vi "GviewerMain.vi"() -> ()   [LabVIEW 2020, in "Gviewer.lvclass"]
doc: "Main Graph Viewer.\nSeveral instances of this viewer can run simultaneously."
uses:
  Gviewer.lvclass
  controls/Typedef_Live.ctl
  Gserver/controls/Typedef_Gviewer-Query.ctl
  Gserver/controls/Typedef_QueryType.ctl
  Gviewer.lvclass/Gviewer.ctl
  FAMM/controls/FAMM_reply_datagram.ctl
  FAMM/controls/FAMM_reply_PAQdata.ctl
  FAMM/controls/FAMM_reply_WAQdata.ctl
  FAMM/controls/FAMM_reply_EAQdata.ctl
  controls/ToolBarAppearance.ctl
  controls/KeyPress.ctl
  <vilib>/event_ctls.llb/eventvkey.ctl
  Gserver/Gserver.lvclass
  FAMM/FAMM.lvclass
panel:
  in  "StartupTagList":string[](array[string])
  in  "Gserver-Queue":refnum<queue>
  in  "GviewName":string="Gview-01"
  in  "Live":T1
  out "ToolBar":picture
  out "Graph":cluster{dbl[], "data":dbl[]}[](graph)
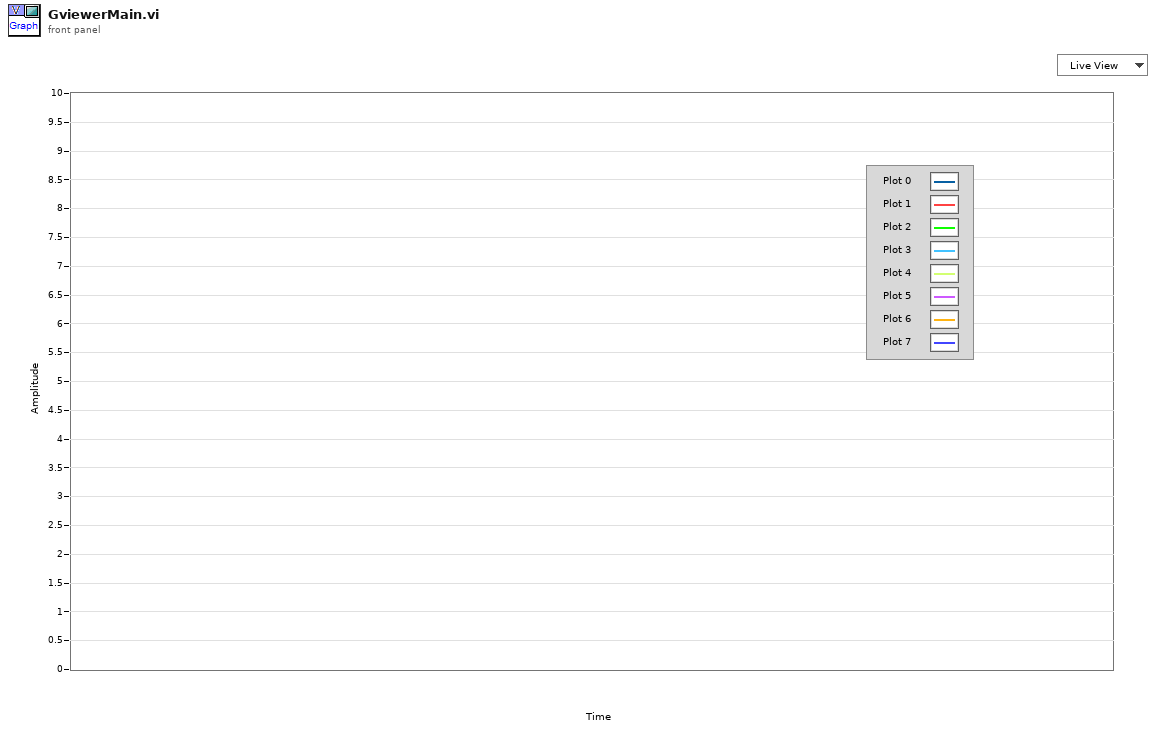
[diagram p1: front panel]
types:
  T1 = typedef "Gviewer.lvclass/Typedef_Live.ctl" = enum16{"Live View", "Freeze"}
  T2 = typedef "FAMM.lvclass/FAMM_reply_datagram.ctl" = cluster{"GraphName":string, "Time-Start":timestamp, "Time-End":timestamp, "TimeSpan":dbl, "Live":T1, "PAQ_section":T3, "WAQ_section":T4, "EAQ_section":T5}
  T3 = typedef "FAMM.lvclass/FAMM_reply_PAQdata.ctl" = cluster{"Tags":string[], "time stamp":timestamp[], "DataSection":cluster{"data":dbl[], "max":dbl[], "min":dbl[], "Status":u32[]}[]}
  T4 = typedef "FAMM.lvclass/FAMM_reply_WAQdata.ctl" = cluster{"Boolean":bool}
  T5 = typedef "FAMM.lvclass/FAMM_reply_EAQdata.ctl" = cluster{"Boolean":bool}
  T6 = typedef "Gserver.lvclass/Typedef_QueryType.ctl" = enum16{"Subscribe", "DataRequest", "RequestAllTags", "RequestIniPath", "FAMMstarted", "SetClientOptions", "GviewerUpdate", "OpenNewGraph", "CloseClient", "CloseAllClients", "Close Gserver"}
  T7 = typedef "Gviewer.lvclass/ToolBarAppearance.ctl" = enum16{"Bare", "Native", "Gradient"}
  T8 = typedef "KeyPress.ctl" = cluster{"Char":i16, "VKey":T9, "Shift":bool, "Ctrl":bool, "Time":timestamp}
  T9 = typedef "eventvkey.ctl" = enum16{"ASCII", "Enter", "Return", "Shift", "Ctrl", "Alt", "Cmd", "Opt", "Caps", "NumLock", "Clear", "Break", "Up", "Down", "Left", "Right", "Insert", "Delete", "Home", "End", "PageUp", "PageDown", "Escape", "Help", "Pause", "ScrollLock", "F1", "F2", "F3", "F4", "F5", "F6", "F7", "F8", "F9", "F10", "F11", "F12", "F13", "F14", "F15", "F16", "F17", "F18", "F19", "F20", "F21", "F22", "F23", "F24", "Play", "VolumeUp", "VolumeDown", "Mute", "Two Byte Char"}
  T10 = typedef "Typedef_Gserver-Replies.ctl" = cluster{"ServerActions":T11, "data":variant, "Source":string, "Time Stamp":timestamp}
  T11 = typedef "Typedef_ServerActions.ctl" = enum16{"GraphUpdate", "SendAllTags", "SendIniPath", "SetGeneralOptions", "ExitGraph"}
  T12 = typedef "SettingsGeneral.ctl" = cluster{"MenuBar_active":bool, "ContextMenu_active":bool}
  T13 = typedef "LVPoint32TypeDef.ctl" = cluster{"Horizontal":i32, "Vertical":i32}
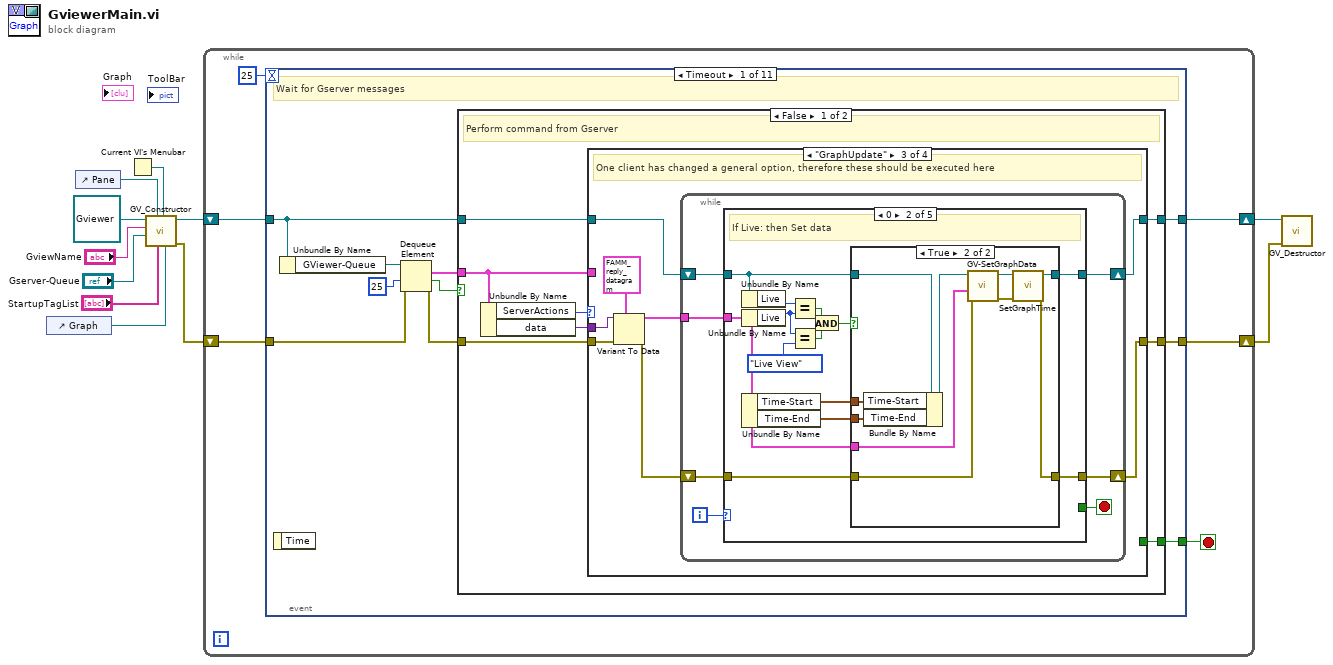
[diagram p0: block diagram]
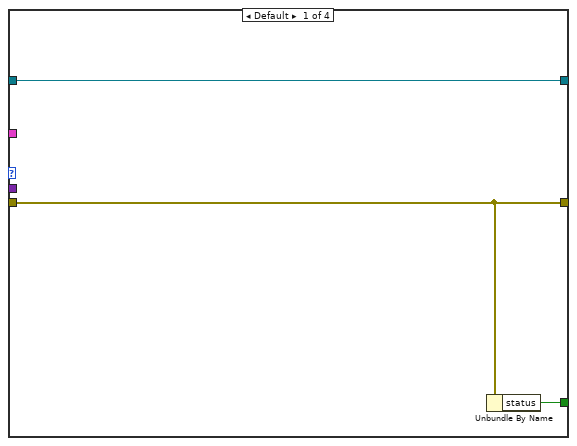
[diagram p2: hidden frame]
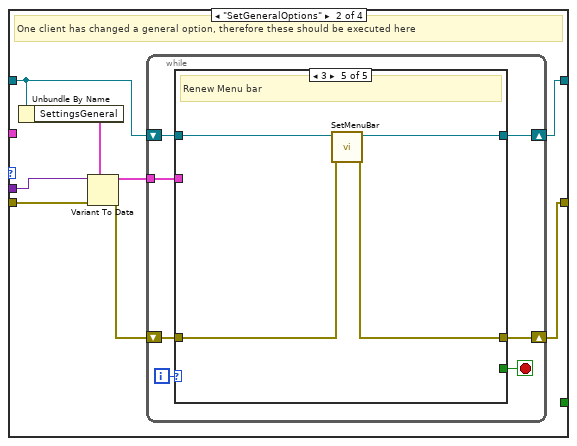
[diagram p3: hidden frame]
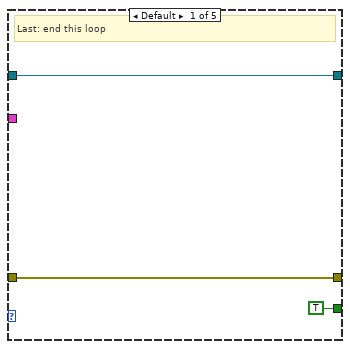
[diagram p4: hidden frame]
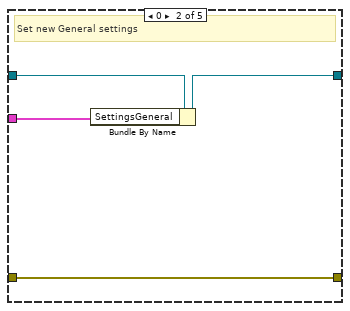
[diagram p5: hidden frame]
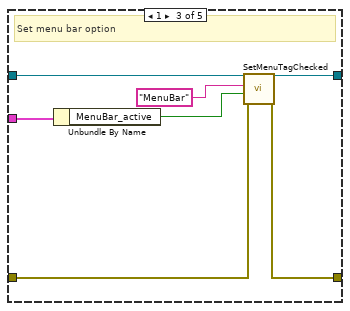
[diagram p6: hidden frame]
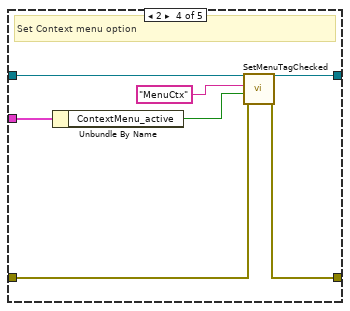
[diagram p7: hidden frame]
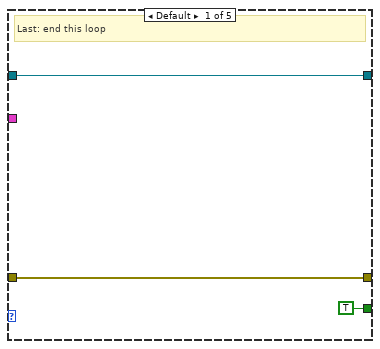
[diagram p8: hidden frame]
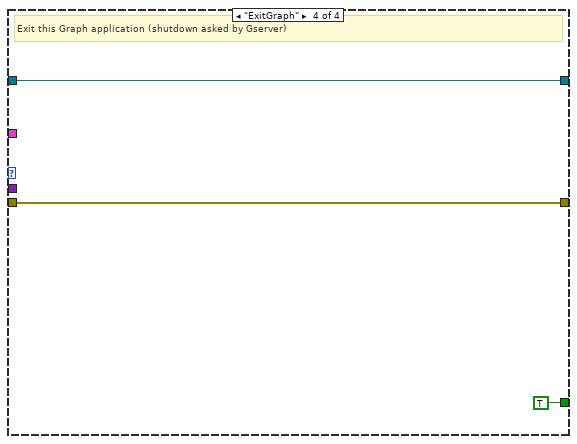
[diagram p13: hidden frame]
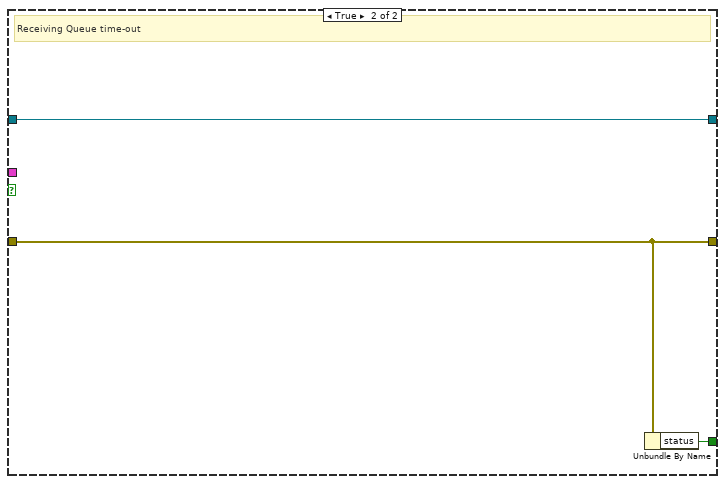
[diagram p14: hidden frame]
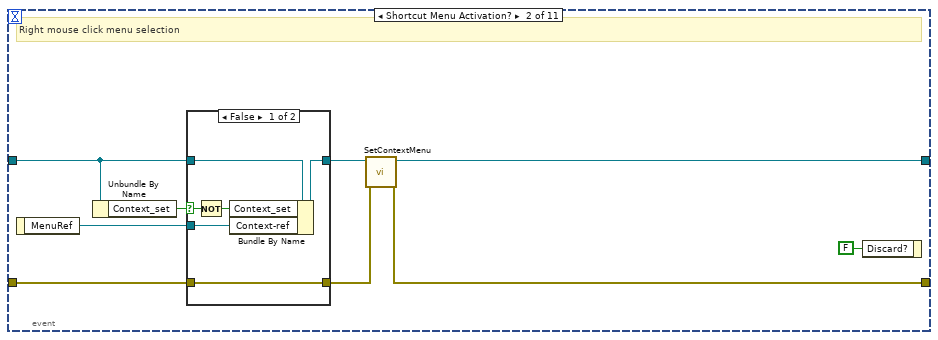
[diagram p15: hidden frame]
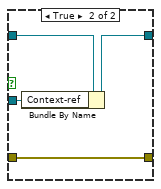
[diagram p16: hidden frame]
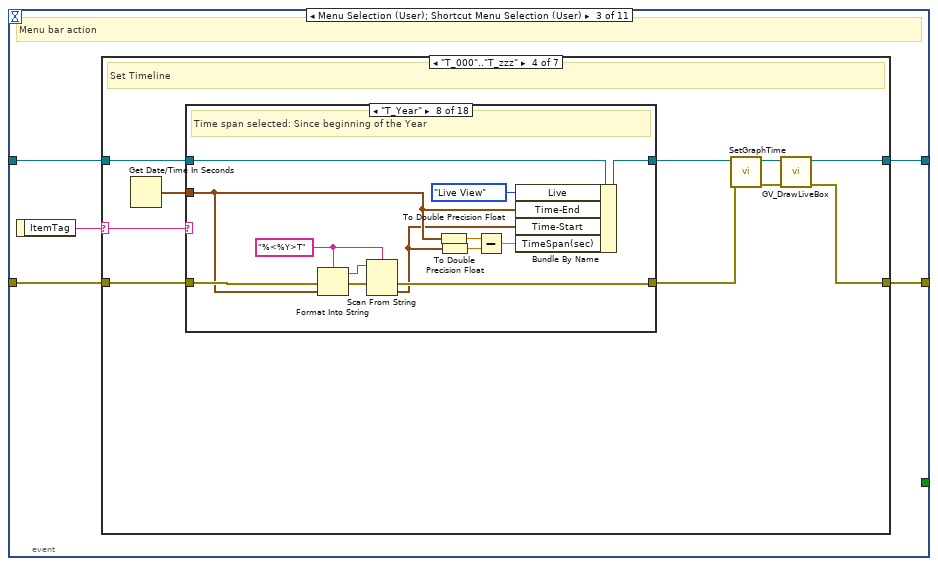
[diagram p17: hidden frame]
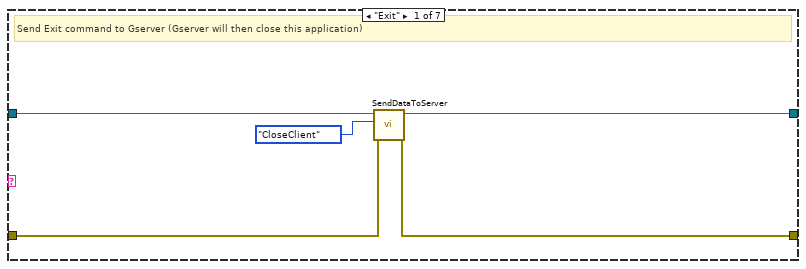
[diagram p18: hidden frame]
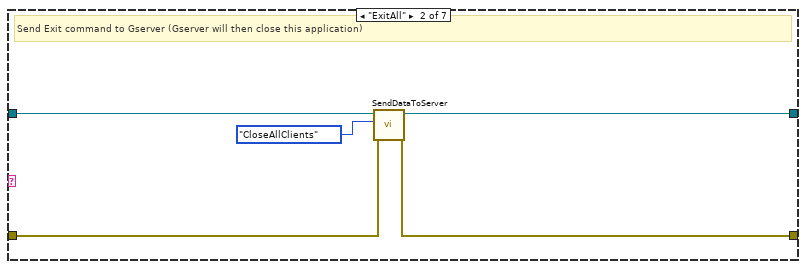
[diagram p19: hidden frame]
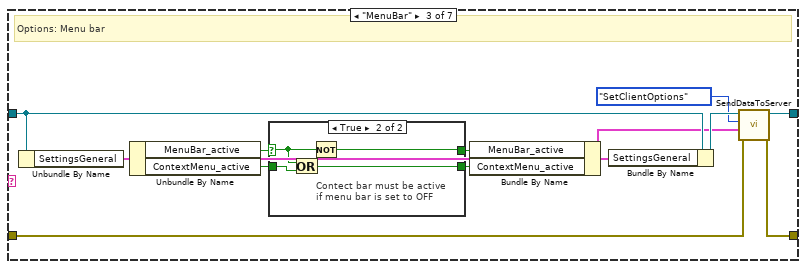
[diagram p20: hidden frame]
diagram:
  n1 = control-ref of="Graph"() -> (w1:refnum<vi>)
  n2 = control-ref of="Pane"() -> (w7:refnum<vi>)
  n3 = Current VI's Menubar() -> (w2:refnum<k9>)
  n4 = call "GV_Constructor.vi"("Graph-ref"=w1, "menu reference"=w2, "StartupTagList"="StartupTagList", "Pane"=w7, "Gserver-Queue"="Gserver-Queue", "GviewName"="GviewName", "Gviewer in"=refnum<class "Gviewer.lvclass"> refnum) -> ("error out"=w3:errorcluster, "Gviewer out"=w10:refnum<class "Gviewer.lvclass">)  [unwired: 3 in]
  n5 = while {
    shift-right: [w15] -> w11
    shift-left: w10 -> [w16]
    shift-right: [w13] -> w9
    shift-left: w3 -> [w14]
    stop <- w12 stop-if-true
    n6 = event shown="[0] Timeout" {
      selector: _ -> [_ _ _ _ _ _ _ _ _ _ _]
      dyn-events: _ -> [_ _ _ _ _ _ _ _ _ _ _]
      timeout: 25 -> [_ _ _ _ _ _ _ _ _ _ _]
      tunnel: w16 -> [w18 w141 w156 w396 w399 w411 w450 w471 w477 w484 w488]
      tunnel: [w21 w135 w154 w391 w397 w406 w444 w472 w475 w481 w487] -> w15
      tunnel: w14 -> [w26 w139 w155 w395 w400 w410 w449 w469 w473 w480 w485]
      tunnel: [w22 w137 w153 w389 w400 w404 w441 w470 w474 w479 w485] -> w13
      tunnel: [w20 _ _ _ _ _ _ _ _ _ _] -> w12
      event Timeout {
        # "Wait for Gserver messages"
        n7 = event-data() -> ()  [unwired: 1 in, 1 out]
        n8 = Unbundle By Name(w18) -> ("GViewer-Queue"=w27:refnum<queue>)
        n9 = Dequeue Element(queue=w27, timeout in ms (-1)=25, error in (no error)=w26) -> (element=w24:T10, timed out?=w19:bool, error out=w23:errorcluster)  [unwired: 1 out]
        n10 = case shown="False" w19 {
          tunnel: w24 -> [w29 _]
          tunnel: w18 -> [w34 w133]
          tunnel: w23 -> [w33 w132]
          tunnel: [w32 w132] -> w22
          tunnel: [w31 w133] -> w21
          tunnel: [w30 w131] -> w20
          frame False {
            # "Perform command from Gserver"
            n11 = Unbundle By Name(w29) -> ("ServerActions"=w35:T11, "data"=w28:variant)
            n12 = case shown="\"GraphUpdate\"" w35 {
              tunnel: w34 -> [w38 w40 w81 w130]
              tunnel: w33 -> [w36 w45 w85 w129]
              tunnel: [w36 w41 w82 w129] -> w32
              tunnel: [w38 w43 w84 w130] -> w31
              tunnel: [w37 _ _ TRUE] -> w30
              tunnel: w29 -> [_ _ _ _]
              tunnel: w28 -> [_ w46 w86 _]
              frame Default {
                n13 = Unbundle By Name(w36) -> ("status"=w37:bool)
              }
              frame "SetGeneralOptions" {
                # "One client has changed a general option, therefore these should be executed here"
                n14 = Unbundle By Name(w40) -> ("SettingsGeneral"=w44:T12)
                n15 = Variant To Data(error in=w45, type=w44, Variant=w46) -> (data=w39:T12, error out=w42:errorcluster)
                n16 = while {
                  shift-right: [w48] -> w43
                  shift-left: w40 -> [w51]
                  shift-right: [w47] -> w41
                  shift-left: w42 -> [w50]
                  tunnel: w39 -> [w49]
                  i -> [w53]
                  stop <- w52 stop-if-true
                  n17 = case shown="3" w53 {
                    tunnel: [TRUE _ _ _ _] -> w52
                    tunnel: w51 -> [w54 w60 w62 w73 w78]
                    tunnel: w50 -> [w55 w57 w64 w69 w76]
                    tunnel: w49 -> [_ w59 w61 w71 _]
                    tunnel: [w54 w58 w66 w72 w77] -> w48
                    tunnel: [w55 w57 w63 w68 w75] -> w47
                    frame Default {
                      # "Last: end this loop"
                    }
                    frame 0 {
                      # "Set new General settings"
                      n18 = Bundle By Name(cluster=w60, "SettingsGeneral"=w59) -> (w58:refnum<class "Gviewer.lvclass">)
                    }
                    frame 1 {
                      # "Set menu bar option"
                      n19 = Unbundle By Name(w61) -> ("MenuBar_active"=w65:bool)
                      n20 = call "SetMenuTagChecked.vi"("error in (no error)"=w64, "Checked"=w65, "TAG"="MenuBar", "Gviewer in"=w62) -> ("error out"=w63:errorcluster, "Gviewer out"=w66:refnum<class "Gviewer.lvclass">)  [unwired: 6 in]
                    }
                    frame 2 {
                      # "Set Context menu option"
                      n21 = Unbundle By Name(w71) -> ("ContextMenu_active"=w70:bool)
                      n22 = call "SetMenuTagChecked.vi"("error in (no error)"=w69, "Checked"=w70, "TAG"="MenuCtx", "Gviewer in"=w73) -> ("error out"=w68:errorcluster, "Gviewer out"=w72:refnum<class "Gviewer.lvclass">)  [unwired: 6 in]
                    }
                    frame 3 {
                      # "Renew Menu bar"
                      n23 = call "SetMenuBar.vi"("error in (no error)"=w76, "Gviewer in"=w78) -> ("error out"=w75:errorcluster, "Gviewer out"=w77:refnum<class "Gviewer.lvclass">)  [unwired: 8 in]
                    }
                  }
                }
              }
              frame "GraphUpdate" {
                # "One client has changed a general option, therefore these should be executed here"
                n24 = Variant To Data(error in=w85, type=T2 {"GraphName"="", "Time-Start"=timestamp(0 s since 1904-01-01), "Time-End"=timestamp(0 s since 1904-01-01), "TimeSpan"=0.0, "Live"=enum."Live View", "PAQ_section"={"Tags"=[], "time stamp"=[], "DataSection"=[]}, "WAQ_section"={"Boolean"=FALSE}, "EAQ_section"={"Boolean"=FALSE}} ("GviewerUpdate"), Variant=w86) -> (data=w80:T2, error out=w83:errorcluster)
                n25 = while {
                  shift-right: [w88] -> w84
                  shift-left: w81 -> [w91]
                  shift-right: [w87] -> w82
                  shift-left: w83 -> [w90]
                  tunnel: w80 -> [w89]
                  i -> [w93]
                  stop <- w92 stop-if-true
                  n26 = case shown="0" w93 {
                    tunnel: [TRUE _ _ _ _] -> w92
                    tunnel: w91 -> [w94 w103 w123 w125 w127]
                    tunnel: w90 -> [w95 w101 w122 w124 w126]
                    tunnel: w89 -> [_ w97 _ _ _]
                    tunnel: [w94 w102 w123 w125 w127] -> w88
                    tunnel: [w95 w100 w122 w124 w126] -> w87
                    frame Default {
                      # "Last: end this loop"
                    }
                    frame 0 {
                      # "If Live: then Set data"
                      n27 = Unbundle By Name(w103) -> ("Live"=w109:T1)
                      n28 = Unbundle By Name(w97) -> ("Live"=w108:T1)
                      n29 = Unbundle By Name(w97) -> ("Time-Start"=w99:timestamp, "Time-End"=w98:timestamp)
                      n30 = Equal?(x=w109, y=w108) -> (x = y?=w106:bool)
                      n31 = Equal?(x=w108, y=Typedef_Live."Live View") -> (x = y?=w105:bool)
                      n32 = And(x=w106, y=w105) -> (x .and. y?=w104:bool)
                      n33 = case shown="True" w104 {
                        tunnel: w103 -> [w111 w119]
                        tunnel: [w111 w118] -> w102
                        tunnel: w101 -> [w110 w113]
                        tunnel: [w110 w117] -> w100
                        tunnel: w99 -> [_ w121]
                        tunnel: w98 -> [_ w120]
                        tunnel: w97 -> [_ w112]
                        frame False {
                        }
                        frame True {
                          n34 = Bundle By Name(cluster=w119, "Time-Start"=w121, "Time-End"=w120) -> (w116:refnum<class "Gviewer.lvclass">)
                          n35 = call "GV-SetGraphData.vi"("error in (no error)"=w113, "GviewerUpdate"=w112, "Gviewer in"=w116) -> ("error out"=w114:errorcluster, "Gviewer out"=w115:refnum<class "Gviewer.lvclass">)  [unwired: 7 in]
                          n36 = call "SetGraphTime.vi"("error in (no error)"=w114, "Gviewer in"=w115) -> ("error out"=w117:errorcluster, "Gviewer out"=w118:refnum<class "Gviewer.lvclass">)  [unwired: 8 in]
                        }
                      }
                    }
                    frame 1 {
                      # "1"
                    }
                    frame 2 {
                      # "2"
                    }
                    frame 3 {
                      # "3"
                    }
                  }
                }
              }
              frame "ExitGraph" {
                # "Exit this Graph application (shutdown asked by Gserver)"
              }
            }
          }
          frame True {
            # "Receiving Queue time-out"
            n37 = Unbundle By Name(w132) -> ("status"=w131:bool)
          }
        }
      }
      event Shortcut Menu Activation? {
        # "Right mouse click menu selection"
        n38 = event-data() -> ("MenuRef"=w140:refnum<k9>)  [unwired: 1 in]
        n39 = Unbundle By Name(w141) -> ("Context_set"=w142:bool)
        n40 = case shown="False" w142 {
          selector: w142 -> [w148 _]
          tunnel: w141 -> [w145 w149]
          tunnel: w140 -> [w146 w151]
          tunnel: w139 -> [w143 w152]
          tunnel: [w143 w152] -> w136
          tunnel: [w144 w150] -> w138
          frame False {
            n41 = Not(x=w148) -> (.not. x?=w147:bool)
            n42 = Bundle By Name(cluster=w145, "Context_set"=w147, "Context-ref"=w146) -> (w144:refnum<class "Gviewer.lvclass">)
          }
          frame True {
            n43 = Bundle By Name(cluster=w149, "Context-ref"=w151) -> (w150:refnum<class "Gviewer.lvclass">)
          }
        }
        n44 = call "SetContextMenu.vi"("error in (no error)"=w136, "Gviewer in"=w138) -> ("error out"=w137:errorcluster, "Gviewer out"=w135:refnum<class "Gviewer.lvclass">)  [unwired: 8 in]
        n45 = event-data("Discard?"=FALSE) -> ()  [unwired: 1 in, 1 out]
      }
      event Menu Selection (User); Shortcut Menu Selection (User) {
        # "Menu bar action"
        n46 = event-data() -> ("ItemTag"=w157:string)  [unwired: 1 in]
        n47 = case shown="\"T_000\"..\"T_zzz\"" w157 {
          selector: w157 -> [_ _ _ w196 _ w377 w387]
          tunnel: w156 -> [w161 w166 w176 w194 w360 w375 w388]
          tunnel: w155 -> [w160 w165 w170 w193 w357 w378 w384]
          tunnel: [w162 w167 w172 w189 w359 w380 w388] -> w154
          tunnel: [w159 w164 w171 w187 w358 w379 w384] -> w153
          frame "Exit" {
            # "Send Exit command to Gserver (Gserver will then close this application)"
            n48 = call "SendDataToServer.vi"("error in (no error)"=w160, "Query_type"=Typedef_QueryType."CloseClient", "Gviewer in"=w161) -> ("error out"=w159:errorcluster, "Gviewer out"=w162:refnum<class "Gviewer.lvclass">)  [unwired: 7 in]
          }
          frame "ExitAll" {
            # "Send Exit command to Gserver (Gserver will then close this application)"
            n49 = call "SendDataToServer.vi"("error in (no error)"=w165, "Query_type"=Typedef_QueryType."CloseAllClients", "Gviewer in"=w166) -> ("error out"=w164:errorcluster, "Gviewer out"=w167:refnum<class "Gviewer.lvclass">)  [unwired: 7 in]
          }
          frame "MenuBar" {
            # "Options: Menu bar"
            n50 = Unbundle By Name(w176) -> ("SettingsGeneral"=w178:T12)
            n51 = Unbundle By Name(w178) -> ("MenuBar_active"=w179:bool, "ContextMenu_active"=w175:bool)
            n52 = case shown="True" w179 {
              selector: w179 -> [w182 w184]
              tunnel: [w181 w186] -> w177
              tunnel: w175 -> [w180 w185]
              tunnel: [w180 w183] -> w174
              frame False {
                n53 = Not(x=w182) -> (.not. x?=w181:bool)
              }
              frame True {
                # "Contect bar must be active\nif menu bar is set to OFF"
                n54 = Or(x=w184, y=w185) -> (x .or. y?=w183:bool)
                n55 = Not(x=w184) -> (.not. x?=w186:bool)
              }
            }
            n56 = Bundle By Name(cluster=w178, "MenuBar_active"=w177, "ContextMenu_active"=w174) -> (w168:T12)
            n57 = Bundle By Name(cluster=w176, "SettingsGeneral"=w168) -> (w173:refnum<class "Gviewer.lvclass">)
            n58 = call "SendDataToServer.vi"("error in (no error)"=w170, "data"=w168, "Query_type"=Typedef_QueryType."SetClientOptions", "Gviewer in"=w173) -> ("error out"=w171:errorcluster, "Gviewer out"=w172:refnum<class "Gviewer.lvclass">)  [unwired: 6 in]
          }
          frame "T_000".."T_zzz" {
            # "Set Timeline"
            n59 = Get Date/Time In Seconds() -> (seconds since 1Jan1904=w195:timestamp)
            n60 = case shown="\"T_Year\"" w196 {
              tunnel: w195 -> [_ _ _ _ _ w236 w249 w262 w275 _ _ _ _ _ _ _ _ _]
              tunnel: w194 -> [w198 w200 w208 w216 w224 w242 w255 w268 w281 w284 w292 w300 w308 w316 w324 w332 w340 w348]
              tunnel: w193 -> [w197 w206 w214 w222 w230 w239 w252 w265 w278 w290 w298 w306 w314 w322 w330 w338 w346 w354]
              tunnel: [w198 w202 w210 w218 w226 w243 w256 w269 w282 w286 w294 w302 w310 w318 w326 w334 w342 w350] -> w192
              tunnel: [w197 w206 w214 w222 w230 w237 w250 w263 w276 w290 w298 w306 w314 w322 w330 w338 w346 w354] -> w191
              frame Default {
                # "Not familiar.. Don't change"
              }
              frame "T_10min" {
                w201 = 600.0  # 10 minutes
                # "Time span selected: 10 minutes"
                n61 = Unbundle By Name(w200) -> ("Time-End"=w199:timestamp)
                n62 = To Double Precision Float(number=w199) -> (double precision float=w205:dbl)
                n63 = Subtract(x=w205, y=w201) -> (x-y=w204:dbl)
                n64 = To Time Stamp(1:w204) -> (0:w203:timestamp)
                n65 = Bundle By Name(cluster=w200, "Time-Start"=w203, "TimeSpan(sec)"=w201) -> (w202:refnum<class "Gviewer.lvclass">)
              }
              frame "T_1hr" {
                w209 = 3600.0  # 60 minutes
                # "Time span selected: 1 hour"
                n66 = Unbundle By Name(w208) -> ("Time-End"=w207:timestamp)
                n67 = To Double Precision Float(number=w207) -> (double precision float=w213:dbl)
                n68 = Subtract(x=w213, y=w209) -> (x-y=w212:dbl)
                n69 = To Time Stamp(1:w212) -> (0:w211:timestamp)
                n70 = Bundle By Name(cluster=w208, "Time-Start"=w211, "TimeSpan(sec)"=w209) -> (w210:refnum<class "Gviewer.lvclass">)
              }
              frame "T_4hr" {
                w217 = 14400.0  # 4 hours
                # "Time span selected: 4 hours"
                n71 = Unbundle By Name(w216) -> ("Time-End"=w215:timestamp)
                n72 = To Double Precision Float(number=w215) -> (double precision float=w221:dbl)
                n73 = Subtract(x=w221, y=w217) -> (x-y=w220:dbl)
                n74 = To Time Stamp(1:w220) -> (0:w219:timestamp)
                n75 = Bundle By Name(cluster=w216, "Time-Start"=w219, "TimeSpan(sec)"=w217) -> (w218:refnum<class "Gviewer.lvclass">)
              }
              frame "T_8hr" {
                w225 = 28800.0  # 8 hours
                # "Time span selected: 4 hours"
                n76 = Unbundle By Name(w224) -> ("Time-End"=w223:timestamp)
                n77 = To Double Precision Float(number=w223) -> (double precision float=w229:dbl)
                n78 = Subtract(x=w229, y=w225) -> (x-y=w228:dbl)
                n79 = To Time Stamp(1:w228) -> (0:w227:timestamp)
                n80 = Bundle By Name(cluster=w224, "Time-Start"=w227, "TimeSpan(sec)"=w225) -> (w226:refnum<class "Gviewer.lvclass">)
              }
              frame "T_Today" {
                w241 = "%<%Y-%j>T" ("format string")
                # "Year + Day number"
                # "Time span selected: Since beginning of Today"
                n81 = Format Into String(format string=w241, error in=w239, w236) -> (resulting string=w240:string, error out=w238:errorcluster)  [unwired: 1 in]
                n82 = Scan From String(format string=w241, input string=w240, error in=w238) -> (error out=w237:errorcluster, output 1=w235:timestamp)  [unwired: 2 in, 2 out]
                n83 = To Double Precision Float(number=w236) -> (double precision float=w233:dbl)
                n84 = To Double Precision Float(number=w235) -> (double precision float=w232:dbl)
                n85 = Subtract(x=w233, y=w232) -> (x-y=w234:dbl)
                n86 = Bundle By Name(cluster=w242, "Live"=Typedef_Live."Live View", "Time-End"=w236, "Time-Start"=w235, "TimeSpan(sec)"=w234) -> (w243:refnum<class "Gviewer.lvclass">)
              }
              frame "T_month" {
                w254 = "%<%Y-%m>T" ("format string")
                # "Year + Month"
                # "Time span selected: Since beginning of this month"
                n87 = Format Into String(format string=w254, error in=w252, w249) -> (resulting string=w253:string, error out=w251:errorcluster)  [unwired: 1 in]
                n88 = Scan From String(format string=w254, input string=w253, error in=w251) -> (error out=w250:errorcluster, output 1=w248:timestamp)  [unwired: 2 in, 2 out]
                n89 = To Double Precision Float(number=w249) -> (double precision float=w246:dbl)
                n90 = To Double Precision Float(number=w248) -> (double precision float=w245:dbl)
                n91 = Subtract(x=w246, y=w245) -> (x-y=w247:dbl)
                n92 = Bundle By Name(cluster=w255, "Live"=Typedef_Live."Live View", "Time-End"=w249, "Time-Start"=w248, "TimeSpan(sec)"=w247) -> (w256:refnum<class "Gviewer.lvclass">)
              }
              frame "T_Year" {
                w267 = "%<%Y>T" ("format string")
                # "Time span selected: Since beginning of the Year"
                n93 = Format Into String(format string=w267, error in=w265, w262) -> (resulting string=w266:string, error out=w264:errorcluster)  [unwired: 1 in]
                n94 = Scan From String(format string=w267, input string=w266, error in=w264) -> (error out=w263:errorcluster, output 1=w261:timestamp)  [unwired: 2 in, 2 out]
                n95 = To Double Precision Float(number=w262) -> (double precision float=w259:dbl)
                n96 = To Double Precision Float(number=w261) -> (double precision float=w258:dbl)
                n97 = Subtract(x=w259, y=w258) -> (x-y=w260:dbl)
                n98 = Bundle By Name(cluster=w268, "Live"=Typedef_Live."Live View", "Time-End"=w262, "Time-Start"=w261, "TimeSpan(sec)"=w260) -> (w269:refnum<class "Gviewer.lvclass">)
              }
              frame "T_Week" {
                w280 = "%<%Y-%W>T" ("format string")
                # "Year + Week number"
                # "Time span selected: since beginning of this week"
                n99 = Format Into String(format string=w280, error in=w278, w275) -> (resulting string=w279:string, error out=w277:errorcluster)  [unwired: 1 in]
                n100 = Scan From String(format string=w280, input string=w279, error in=w277) -> (error out=w276:errorcluster, output 1=w274:timestamp)  [unwired: 2 in, 2 out]
                n101 = To Double Precision Float(number=w275) -> (double precision float=w272:dbl)
                n102 = To Double Precision Float(number=w274) -> (double precision float=w271:dbl)
                n103 = Subtract(x=w272, y=w271) -> (x-y=w273:dbl)
                n104 = Bundle By Name(cluster=w281, "Live"=Typedef_Live."Live View", "Time-End"=w275, "Time-Start"=w274, "TimeSpan(sec)"=w273) -> (w282:refnum<class "Gviewer.lvclass">)
              }
              frame "T_1day" {
                w285 = 86400.0  # 1 day
                # "Time span selected: 1 day"
                n105 = Unbundle By Name(w284) -> ("Time-End"=w283:timestamp)
                n106 = To Double Precision Float(number=w283) -> (double precision float=w289:dbl)
                n107 = Subtract(x=w289, y=w285) -> (x-y=w288:dbl)
                n108 = To Time Stamp(1:w288) -> (0:w287:timestamp)
                n109 = Bundle By Name(cluster=w284, "Time-Start"=w287, "TimeSpan(sec)"=w285) -> (w286:refnum<class "Gviewer.lvclass">)
              }
              frame "T_2days" {
                w293 = 172800.0  # 2 days
                # "Time span selected: 2 days"
                n110 = Unbundle By Name(w292) -> ("Time-End"=w291:timestamp)
                n111 = To Double Precision Float(number=w291) -> (double precision float=w297:dbl)
                n112 = Subtract(x=w297, y=w293) -> (x-y=w296:dbl)
                n113 = To Time Stamp(1:w296) -> (0:w295:timestamp)
                n114 = Bundle By Name(cluster=w292, "Time-Start"=w295, "TimeSpan(sec)"=w293) -> (w294:refnum<class "Gviewer.lvclass">)
              }
              frame "T_5days" {
                w301 = 432000.0  # 5 days
                # "Time span selected: 5 days"
                n115 = Unbundle By Name(w300) -> ("Time-End"=w299:timestamp)
                n116 = To Double Precision Float(number=w299) -> (double precision float=w305:dbl)
                n117 = Subtract(x=w305, y=w301) -> (x-y=w304:dbl)
                n118 = To Time Stamp(1:w304) -> (0:w303:timestamp)
                n119 = Bundle By Name(cluster=w300, "Time-Start"=w303, "TimeSpan(sec)"=w301) -> (w302:refnum<class "Gviewer.lvclass">)
              }
              frame "T_1wk" {
                w309 = 604800.0  # 7 days
                # "Time span selected: 1 week"
                n120 = Unbundle By Name(w308) -> ("Time-End"=w307:timestamp)
                n121 = To Double Precision Float(number=w307) -> (double precision float=w313:dbl)
                n122 = Subtract(x=w313, y=w309) -> (x-y=w312:dbl)
                n123 = To Time Stamp(1:w312) -> (0:w311:timestamp)
                n124 = Bundle By Name(cluster=w308, "Time-Start"=w311, "TimeSpan(sec)"=w309) -> (w310:refnum<class "Gviewer.lvclass">)
              }
              frame "T_2wks" {
                w317 = 1209600.0  # 14 days
                # "Time span selected: 2 weeks"
                n125 = Unbundle By Name(w316) -> ("Time-End"=w315:timestamp)
                n126 = To Double Precision Float(number=w315) -> (double precision float=w321:dbl)
                n127 = Subtract(x=w321, y=w317) -> (x-y=w320:dbl)
                n128 = To Time Stamp(1:w320) -> (0:w319:timestamp)
                n129 = Bundle By Name(cluster=w316, "Time-Start"=w319, "TimeSpan(sec)"=w317) -> (w318:refnum<class "Gviewer.lvclass">)
              }
              frame "T_1month" {
                w325 = 2678400.0  # 31 days
                # "Time span selected: one month"
                n130 = Unbundle By Name(w324) -> ("Time-End"=w323:timestamp)
                n131 = To Double Precision Float(number=w323) -> (double precision float=w329:dbl)
                n132 = Subtract(x=w329, y=w325) -> (x-y=w328:dbl)
                n133 = To Time Stamp(1:w328) -> (0:w327:timestamp)
                n134 = Bundle By Name(cluster=w324, "Time-Start"=w327, "TimeSpan(sec)"=w325) -> (w326:refnum<class "Gviewer.lvclass">)
              }
              frame "T_3months" {
                w333 = 7948800.0  # 92 days
                # "Time span selected: 1/4 Year"
                n135 = Unbundle By Name(w332) -> ("Time-End"=w331:timestamp)
                n136 = To Double Precision Float(number=w331) -> (double precision float=w337:dbl)
                n137 = Subtract(x=w337, y=w333) -> (x-y=w336:dbl)
                n138 = To Time Stamp(1:w336) -> (0:w335:timestamp)
                n139 = Bundle By Name(cluster=w332, "Time-Start"=w335, "TimeSpan(sec)"=w333) -> (w334:refnum<class "Gviewer.lvclass">)
              }
              frame "T_6months" {
                w341 = 15811200.0  # 183 days
                # "Time span selected: 1/2 Year"
                n140 = Unbundle By Name(w340) -> ("Time-End"=w339:timestamp)
                n141 = To Double Precision Float(number=w339) -> (double precision float=w345:dbl)
                n142 = Subtract(x=w345, y=w341) -> (x-y=w344:dbl)
                n143 = To Time Stamp(1:w344) -> (0:w343:timestamp)
                n144 = Bundle By Name(cluster=w340, "Time-Start"=w343, "TimeSpan(sec)"=w341) -> (w342:refnum<class "Gviewer.lvclass">)
              }
              frame "T_1year" {
                w349 = 31536000.0  # 365 days
                # "Time span selected: one Year"
                n145 = Unbundle By Name(w348) -> ("Time-End"=w347:timestamp)
                n146 = To Double Precision Float(number=w347) -> (double precision float=w353:dbl)
                n147 = Subtract(x=w353, y=w349) -> (x-y=w352:dbl)
                n148 = To Time Stamp(1:w352) -> (0:w351:timestamp)
                n149 = Bundle By Name(cluster=w348, "Time-Start"=w351, "TimeSpan(sec)"=w349) -> (w350:refnum<class "Gviewer.lvclass">)
              }
            }
            n150 = call "SetGraphTime.vi"("error in (no error)"=w191, "Gviewer in"=w192) -> ("error out"=w188:errorcluster, "Gviewer out"=w190:refnum<class "Gviewer.lvclass">)  [unwired: 8 in]
            n151 = call "GV_DrawLiveBox.vi"("error in (no error)"=w188, "Gviewer in"=w190) -> ("error out"=w187:errorcluster, "Gviewer out"=w189:refnum<class "Gviewer.lvclass">)  [unwired: 8 in]
          }
          frame "MenuCtx" {
            # "Options: Context menu"
            n152 = Unbundle By Name(w360) -> ("SettingsGeneral"=w365:T12)
            n153 = Unbundle By Name(w365) -> ("ContextMenu_active"=w366:bool, "MenuBar_active"=w363:bool)
            n154 = case shown="True" w366 {
              selector: w366 -> [w369 w371]
              tunnel: [w368 w373] -> w364
              tunnel: w363 -> [w367 w372]
              tunnel: [w367 w370] -> w362
              frame False {
                n155 = Not(x=w369) -> (.not. x?=w368:bool)
              }
              frame True {
                # "menu bar must be active\nif context menu is set to OFF"
                n156 = Or(x=w371, y=w372) -> (x .or. y?=w370:bool)
                n157 = Not(x=w371) -> (.not. x?=w373:bool)
              }
            }
            n158 = Bundle By Name(cluster=w365, "ContextMenu_active"=w364, "MenuBar_active"=w362) -> (w356:T12)
            n159 = Bundle By Name(cluster=w360, "SettingsGeneral"=w356) -> (w355:refnum<class "Gviewer.lvclass">)
            n160 = call "SendDataToServer.vi"("error in (no error)"=w357, "data"=w356, "Query_type"=Typedef_QueryType."SetClientOptions", "Gviewer in"=w355) -> ("error out"=w358:errorcluster, "Gviewer out"=w359:refnum<class "Gviewer.lvclass">)  [unwired: 6 in]
          }
          frame "ToolBare", "ToolGradient", "ToolNative" {
            # "Toolbar appearance layout change"
            n161 = case shown="\"ToolGradient\"" w377 {
              tunnel: [ToolBarAppearance."Native" ("ToolBarAppearance") ToolBarAppearance."Bare" ("ToolBarAppearance") ToolBarAppearance."Gradient" ("ToolBarAppearance")] -> w374
              frame Default {
              }
              frame "ToolBare" {
              }
              frame "ToolGradient" {
              }
            }
            n162 = Bundle By Name(cluster=w375, "ToolBarAppearance"=w374) -> (w376:refnum<class "Gviewer.lvclass">)
            n163 = call "GV_SetToolbar.vi"("error in (no error)"=w378, "Gviewer in"=w376) -> ("error out"=w379:errorcluster, "Gviewer out"=w380:refnum<class "Gviewer.lvclass">)  [unwired: 8 in]
          }
          frame Default {
            n164 = Concatenate Strings("Menu item not implemented:\n", w387) -> (w386:string)
            n165 = One Button Dialog(message=w386) -> ()  [unwired: 1 in, 1 out]
          }
        }
      }
      event Pane Size {
        # "Rearange all objects to Pane size"
        n166 = event-data() -> ()  [unwired: 1 in, 3 out]
        n167 = call "GV_SetToolbar.vi"("error in (no error)"=w395, "Gviewer in"=w396) -> ("error out"=w393:errorcluster, "Gviewer out"=w394:refnum<class "Gviewer.lvclass">)  [unwired: 8 in]
        n168 = call "GV_SetGraph.vi"("error in (no error)"=w393, "Gviewer in"=w394) -> ("error out"=w390:errorcluster, "Gviewer out"=w392:refnum<class "Gviewer.lvclass">)  [unwired: 8 in]
        n169 = call "GV_DrawLiveBox.vi"("error in (no error)"=w390, "Gviewer in"=w392) -> ("error out"=w389:errorcluster, "Gviewer out"=w391:refnum<class "Gviewer.lvclass">)  [unwired: 8 in]
      }
      event "Graph": Mouse Move {
        # "Draw cursor info when mouse is moved"
        n170 = event-data() -> ("Coords"=w398:T13)  [unwired: 1 in]
        n171 = call "CursorDraw.vi"("Coords"=w398, "Gviewer in"=w399) -> ("Gviewer out"=w397:refnum<class "Gviewer.lvclass">)  [unwired: 8 in, 1 out]
      }
      event Key Down {
        # "Press a key"
        n172 = event-data() -> ("ScanCode"=w408:i16, "VKey"=w416:T9, "PlatMods.Shift"=w415:bool, "PlatMods.Ctrl"=w414:bool)  [unwired: 1 in]
        n173 = Unbundle By Name(w411) -> ("KeyStrokes_Lookup"=w418:i16[])
        n174 = Get Date/Time In Seconds() -> (seconds since 1Jan1904=w413:timestamp)
        n175 = Search 1D Array(1D array=w418, element=w408) -> (index of element=w412:i32)  [unwired: 1 in]
        n176 = Bundle By Name(cluster=T8 {"Char"=0, "VKey"=enum."ASCII", "Shift"=FALSE, "Ctrl"=FALSE, "Time"=timestamp(0 s since 1904-01-01)} ("Key"), "Char"=w408, "VKey"=w416, "Shift"=w415, "Ctrl"=w414, "Time"=w413) -> (w409:T8)
        n177 = case shown="Default" w412 {
          selector: w412 -> [w425 _]
          tunnel: w411 -> [w419 w439]
          tunnel: w410 -> [w428 w430]
          tunnel: [w428 w431] -> w407
          tunnel: [w420 w432] -> w402
          tunnel: w409 -> [w424 w429]
          tunnel: w408 -> [w423 w436]
          frame Default {
            # "Replace if the switch action already exists"
            n178 = Unbundle By Name(w419) -> ("KeyStrokes_Lookup"=w427:i16[], "KeyStrokes"=w426:T8[])
            n179 = Replace Array Subset(array=w427, new element=w423, index=w425) -> (w422:i16[])
            n180 = Replace Array Subset(array=w426, new element=w424, index=w425) -> (w421:T8[])
            n181 = Bundle By Name(cluster=w419, "KeyStrokes_Lookup"=w422, "KeyStrokes"=w421) -> (w420:refnum<class "Gviewer.lvclass">)
          }
          frame -1 {
            # "Actions on switch pressing\nare in here"
            # "New switch pressure"
            n182 = Unbundle By Name(w439) -> ("KeyStrokes_Lookup"=w438:i16[], "KeyStrokes"=w435:T8[])
            n183 = Build Array (concatenate)(w435, w429) -> (w434:T8[])
            n184 = Build Array (concatenate)(w438, w436) -> (w437:i16[])
            n185 = Bundle By Name(cluster=w439, "KeyStrokes_Lookup"=w437, "KeyStrokes"=w434) -> (w433:refnum<class "Gviewer.lvclass">)
            n186 = call "KeySwitched.vi"("error in (no error)"=w430, "Key"=w429, "Gviewer in"=w433) -> ("error out"=w431:errorcluster, "Gviewer out"=w432:refnum<class "Gviewer.lvclass">)  [unwired: 7 in]
          }
        }
        n187 = Unbundle By Name(w402) -> ("GraphCursorLoc"=w401:T13)
        n188 = call "ToolBarButtonDraw.vi"("error in (no error)"=w407, "Gviewer in"=w402) -> ("error out"=w405:errorcluster, "Gviewer out"=w403:refnum<class "Gviewer.lvclass">)  [unwired: 8 in]
        n189 = call "CursorDraw.vi"("error in (no error)"=w405, "Coords"=w401, "Gviewer in"=w403) -> ("error out"=w404:errorcluster, "Gviewer out"=w406:refnum<class "Gviewer.lvclass">)  [unwired: 7 in]
      }
      event Key Up {
        # "Release a key"
        n190 = event-data() -> ("ScanCode"=w447:i16)  [unwired: 1 in]
        n191 = Unbundle By Name(w450) -> ("KeyStrokes_Lookup"=w448:i16[])
        n192 = Search 1D Array(1D array=w448, element=w447) -> (index of element=w451:i32)  [unwired: 1 in]
        n193 = case shown="Default" w451 {
          selector: w451 -> [w460 _]
          tunnel: w450 -> [w461 w467]
          tunnel: w449 -> [w453 w466]
          tunnel: [w458 w467] -> w440
          tunnel: [w454 w466] -> w442
          frame Default {
            w456 = 1 ("index")
            n194 = Unbundle By Name(w461) -> ("KeyStrokes_Lookup"=w465:i16[], "KeyStrokes"=w464:T8[])
            n195 = Delete From Array(array=w465, length=w456, index=w460) -> (array with subset deleted=w463:i16[])  [unwired: 1 out]
            n196 = Delete From Array(array=w464, length=w456, index=w460) -> (deleted portion=w457:T8[], array with subset deleted=w462:T8[])
            n197 = Bundle By Name(cluster=w461, "KeyStrokes_Lookup"=w463, "KeyStrokes"=w462) -> (w459:refnum<class "Gviewer.lvclass">)
            n198 = Index Array(array=w457, index=0) -> (element=w455:T8)
            n199 = call "KeyUnSwitched.vi"("error in (no error)"=w453, "Key"=w455, "Gviewer in"=w459) -> ("error out"=w454:errorcluster, "Gviewer out"=w458:refnum<class "Gviewer.lvclass">)  [unwired: 7 in]
          }
          frame -1 {
          }
        }
        n200 = Unbundle By Name(w440) -> ("GraphCursorLoc"=w445:T13)
        n201 = call "ToolBarButtonDraw.vi"("error in (no error)"=w442, "Gviewer in"=w440) -> ("error out"=w443:errorcluster, "Gviewer out"=w446:refnum<class "Gviewer.lvclass">)  [unwired: 8 in]
        n202 = call "CursorDraw.vi"("error in (no error)"=w443, "Coords"=w445, "Gviewer in"=w446) -> ("error out"=w441:errorcluster, "Gviewer out"=w444:refnum<class "Gviewer.lvclass">)  [unwired: 7 in]
      }
      event "ToolBar": Mouse Move {
        # "Update toolbar icons when hovering over it"
        n203 = event-data() -> ("Coords"=w468:T13)  [unwired: 1 in]
        n204 = call "ToolBarButtonDraw.vi"("error in (no error)"=w469, "Coords"=w468, "Gviewer in"=w471) -> ("error out"=w470:errorcluster, "Gviewer out"=w472:refnum<class "Gviewer.lvclass">)  [unwired: 7 in]
      }
      event "ToolBar": Mouse Down {
        # "Press a button on the toolbar"
        n205 = event-data() -> ()  [unwired: 1 in, 2 out]
        n206 = Unbundle By Name(w477) -> ("ToolButtonFocus"=w478:i32)
        n207 = Bundle By Name(cluster=w477, "ToolButtonSelected"=w478) -> (w476:refnum<class "Gviewer.lvclass">)
        n208 = call "ToolBarButtonDraw.vi"("error in (no error)"=w473, "Gviewer in"=w476) -> ("error out"=w474:errorcluster, "Gviewer out"=w475:refnum<class "Gviewer.lvclass">)  [unwired: 8 in]
      }
      event Value Change {
        # "Set Graph mode to 'live' (continous updates)"
        n209 = event-data() -> ("NewVal"=w483:T1)  [unwired: 1 in]
        n210 = Bundle By Name(cluster=w484, "Live"=w483) -> (w482:refnum<class "Gviewer.lvclass">)
        n211 = call "GV_DrawLiveBox.vi"("error in (no error)"=w480, "Gviewer in"=w482) -> ("error out"=w479:errorcluster, "Gviewer out"=w481:refnum<class "Gviewer.lvclass">)  [unwired: 8 in]
      }
      event Panel Close? {
        # "On closing action of this Graph: Ask the Gserver to perform the closing (to ensure that reference in Gserver is removed)"
        n212 = event-data() -> ()  [unwired: 1 in, 4 out]
        n213 = call "SendDataToServer.vi"("Query_type"=Typedef_QueryType."CloseClient", "Gviewer in"=w488) -> ("Gviewer out"=w487:refnum<class "Gviewer.lvclass">)  [unwired: 8 in, 1 out]
        n214 = event-data("Discard?"=TRUE) -> ()  [unwired: 1 in, 1 out]
      }
    }
  }
  n215 = call "GV_Destructor.vi"("error in (no error)"=w9, "Gviewer in"=w11) -> ()  [unwired: 8 in, 2 out]
